vi "NI9623_SUB-VI_GenerateRampWave.vi"(8 "error in (no error)":errorcluster, 9 "sampling info":cluster{"Fs":dbl, "#s":dbl}={"Fs"=1000.0, "#s"=1000.0} {"Fs" format="%.2p"}, 10 "End":dbl=1.0 format="%0.2p", 11 "Start":dbl format="%0.2p") -> (0 "error out":errorcluster, 3 "signal out":waveform(dbl))   [LabVIEW 2020]
uses:
  <vilib>/measure/NI_MABase.lvlib
panel:
  out "Freq(Hz)":dbl
  out "Waveform Graph":waveform(dbl)(graph)
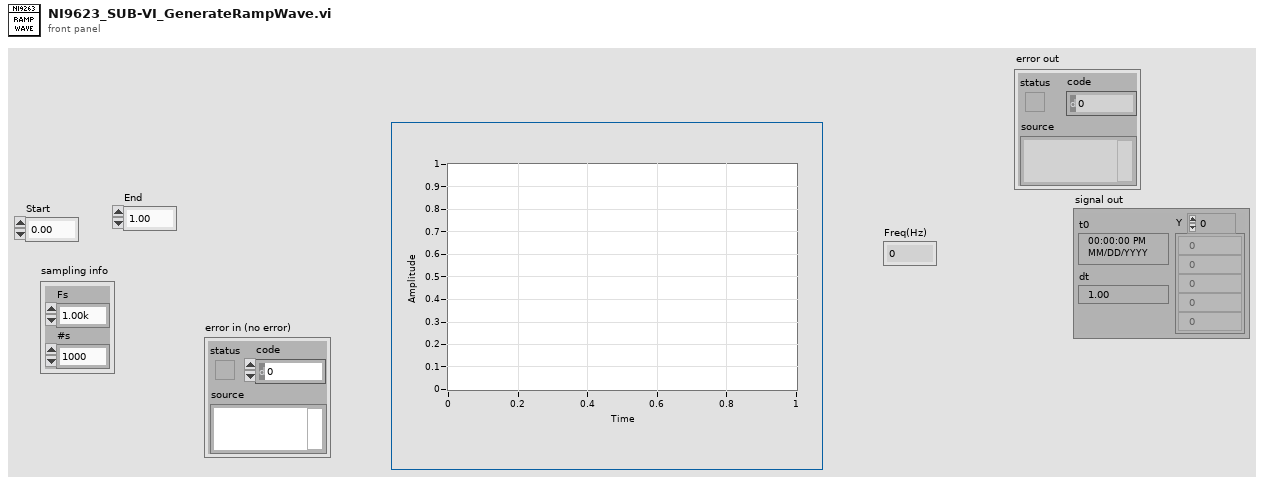
[diagram p1: front panel]
types:
  T1 = enum16{"Sine Wave", "Triangle Wave", "Square Wave", "Sawtooth Wave"}
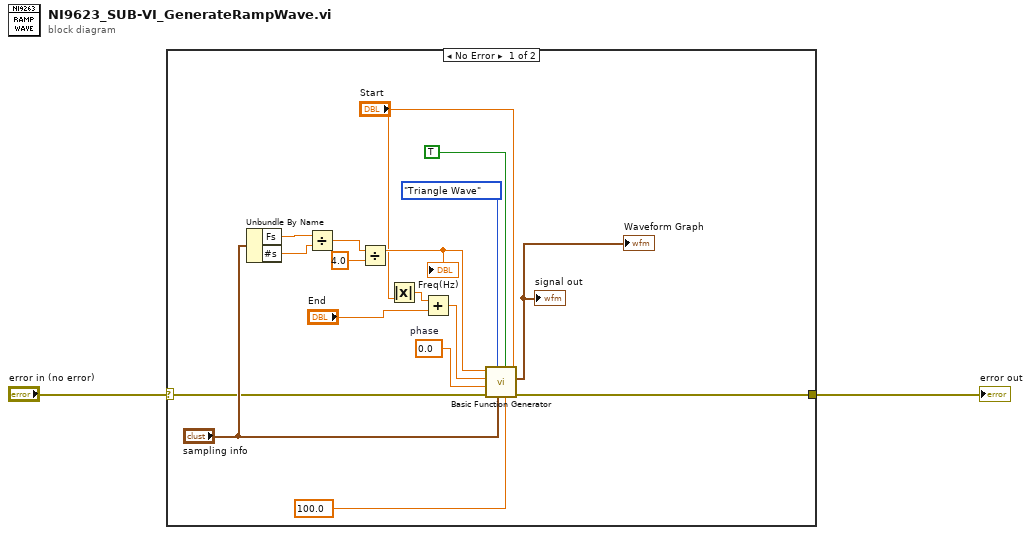
[diagram p0: block diagram]
diagram:
  n1 = case shown="No Error" "error in (no error)" {
    selector: "error in (no error)" -> [w3 w20]
    tunnel: [w15 w20] -> w2
    frame No Error {
      w16 = 0.0  # phase
      n2 = Unbundle By Name("sampling info") -> ("Fs"=w12:dbl, "#s"=w11:dbl)
      n3 = Divide(x=w12, y=w11) -> (x/y=w10:dbl)
      n4 = Divide(x=w10, y=4.0) -> (x/y=w8:dbl)
      "Freq(Hz)" <- w8
      n5 = Absolute Value(x="Start") -> (abs(x)=w4:dbl)
      n6 = Add(x=w4, y="End") -> (x+y=w5:dbl)
      n7 = call <vilib>:"Basic Function Generator.vi"("offset"="Start", "square wave duty cycle (%)"=100.0, "reset signal"=TRUE, "sampling info"="sampling info", "signal type"=T1."Triangle Wave", "error in (no error)"=w3, "phase"=w16, "amplitude"=w5, "frequency"=w8) -> ("error out"=w15:errorcluster, "signal out"=→"signal out" →"Waveform Graph":waveform(dbl))  [unwired: 1 out]
    }
    frame Error {
    }
  }
  "error out" <- w2
